vi "CRC16CHECK.vi"(11 "buf":u8[](array[numeric])) -> (0 "CRCLo":u8, 3 "CRCHi":u8)   [LabVIEW 2015]
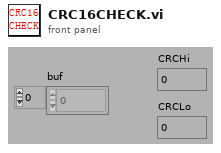
[diagram p1: front panel]
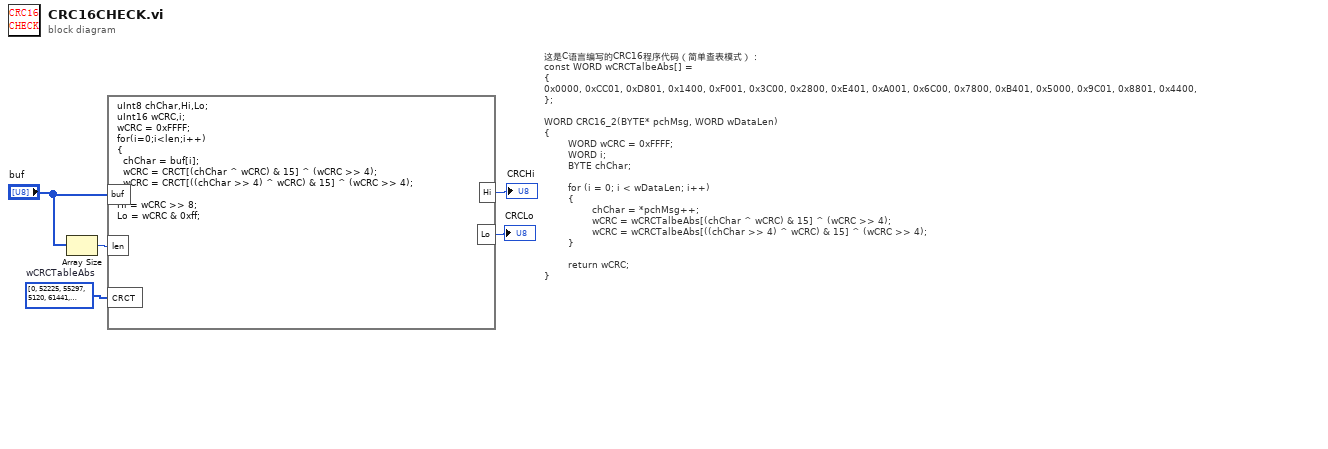
[diagram p0: block diagram]
diagram:
  w5 = u16[] [0, 52225, 55297, 5120, 61441, 15360, 10240, 58369, 40961, 27648, 30720, 46081, 20480, 39937, 34817, 17408]  # wCRCTableAbs
  # "这是C语言编写的CRC16程序代码（简单查表模式）：\nconst WORD wCRCTalbeAbs[] =\n{\n0x0000, 0xCC01, 0xD801, 0x1400, 0xF001, 0x3C00, 0x2800, 0xE401, 0xA001, 0x6C00, 0x7800, 0xB401, 0x5000, 0x9C01, 0x8801, 0x4400, \n};\n\nWORD CRC16_2(BYTE* pchMsg, WORD wDataLen)\n{\n        WORD wCRC = 0xFFFF;\n        WORD i;\n        BYTE chChar;\n\n        for (i = 0; i < wDataLen; i++)\n        {\n                chChar = *pchMsg++;\n                wCRC = wCRCTalbeAbs[(chChar ^ wCRC) & 15] ^ (wCRC >> 4);\n                wCRC = wCRCTalbeAbs[((chChar >> 4) ^ wCRC) & 15] ^ (wCRC >> 4);\n        }\n\n        return wCRC;\n}"
  n1 = Array Size(array="buf") -> (size(s)=w4:i32)
  n2 = formula code="uInt8 chChar,Hi,Lo;\nuInt16 wCRC,i;\nwCRC = 0xFFFF;\nfor(i=0;i<len;i++)\n{\n  chChar = buf[i];\n  wCRC = CRCT[(chChar ^ wCRC) & 15] ^ (wCRC >> 4);\n  wCRC = CRCT[((chChar >> 4) ^ wCRC) & 15] ^ (wCRC >> 4);\n}\nHi = wCRC >> 8;\nLo = wCRC & 0xff;"("buf"="buf", "len"=w4, "CRCT"=w5) -> ("Hi"=→"CRCHi":u8, "Lo"=→"CRCLo":u8)
